vi "Error_IN.vi"() -> ()   [LabVIEW 2016]
panel:
  out "Triangle":dynamicdata(graph)
  out "Sine":dynamicdata(graph)
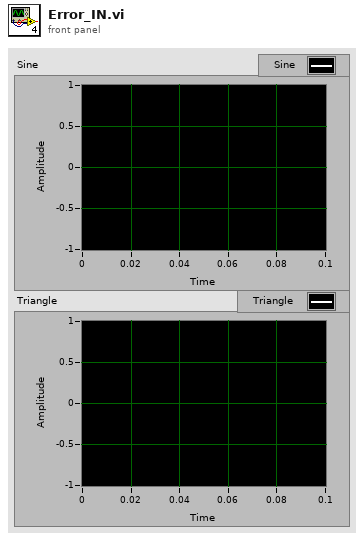
[diagram p1: front panel]
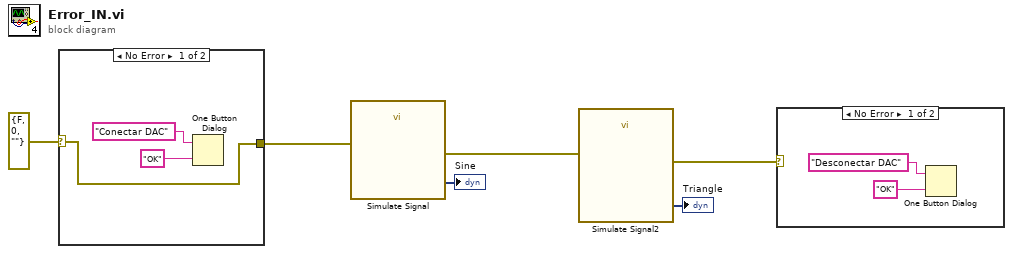
[diagram p0: block diagram]
diagram:
  n1 = case shown="No Error" errorcluster {"status"=FALSE, "code"=0, "source"=""} ("error in (no error)") {
    selector: errorcluster {"status"=FALSE, "code"=0, "source"=""} ("error in (no error)") -> [w7 w10]
    tunnel: [w7 w10] -> w3
    frame No Error {
      n2 = One Button Dialog(message="Conectar DAC", button name ("OK")="OK") -> ()  [unwired: 1 out]
    }
    frame Error {
    }
  }
  n3 = call "Simulate Signal"("error in (no error)"=w3) -> ("Sine"=→"Sine":dynamicdata, "error out"=w2:errorcluster)  [unwired: 13 in]
  n4 = call "Simulate Signal2"("error in (no error)"=w2) -> ("Triangle"=→"Triangle":dynamicdata, "error out"=w1:errorcluster)  [unwired: 13 in]
  n5 = case shown="No Error" w1 {
    frame No Error {
      n6 = One Button Dialog(message="Desconectar DAC", button name ("OK")="OK") -> ()  [unwired: 1 out]
    }
    frame Error {
    }
  }
